vi "sandbox.vi"() -> ()   [LabVIEW 2019, in "Instrument.Lockin.lvlib" / "Instrument UI.Lockin.lvclass"]
uses:
  Instrument UI.Lockin.lvclass
  Instrument.DAQ/Typedefs/State--enum.ctl
  Instrument.DAQ/Instrument.DAQ.lvclass
panel:
  in  "stop":bool
  out "Status":string="Shutdown"
  in  "Enum":T1(ring)=enum."Spinner 3"
  out "delimited string":string
  out "output 1":T2
  # "spinner 3: sweep"
  # "spinner 4: started"
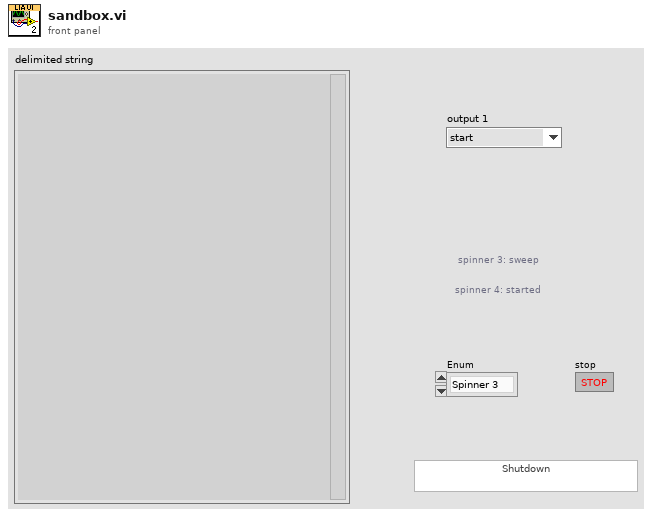
[diagram p1: front panel]
types:
  T1 = enum16{"Spinner 1", "Spinner 2", "Spinner 3", "Spinner 4", "Spinner 5", "Spinner 6"}
  T2 = typedef "Instrument.Lockin.lvlib/Instrument.DAQ.lvclass/State--enum.ctl" = enum16{"start", "stop", "reset", "start sweep", "stop sweep"}
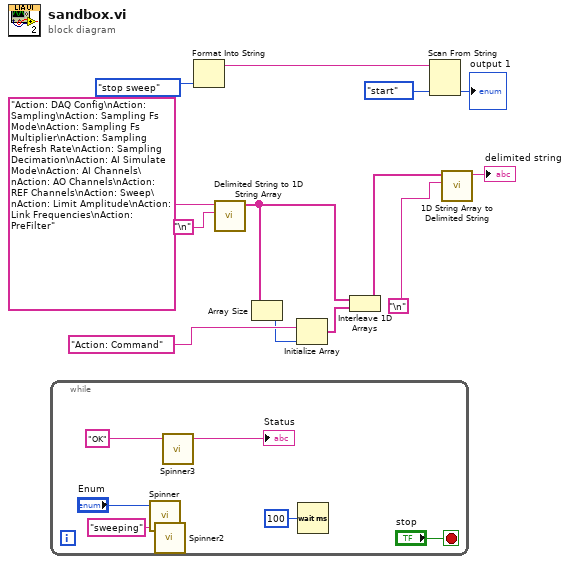
[diagram p0: block diagram]
diagram:
  n1 = while {
    stop <- "stop" stop-if-true
    n2 = call "Spinner.vi"("Enum"="Enum") -> ()  [unwired: 4 in, 1 out]
    n3 = call "Spinner2.vi"("String In"="sweeping") -> ()  [unwired: 4 in, 1 out]
    n4 = call "Spinner3.vi"("String In"="OK") -> ("Spinner Out"=→"Status":string)  [unwired: 4 in]
    n5 = Wait (ms)(milliseconds to wait=u32 100) -> ()  [unwired: 1 out]
  }
  n6 = Format Into String(State--enum."stop sweep" ("State")) -> (resulting string=w11:string)  [unwired: 3 in, 1 out]
  n7 = call <vilib>:"Delimited String to 1D String Array.vi"("delimiter"="\n", "delimited string"="Action: DAQ Config\nAction: Sampling\nAction: Sampling Fs Mode\nAction: Sampling Fs Multiplier\nAction: Sampling Refresh Rate\nAction: Sampling Decimation\nAction: AI Simulate Mode\nAction: AI Channels\nAction: AO Channels\nAction: REF Channels\nAction: Sweep\nAction: Limit Amplitude\nAction: Link Frequencies\nAction: PreFilter" ("State(s) in Front (\"\")")) -> ("string array"=w3:string[])  [unwired: 9 in]
  n8 = Array Size(array=w3) -> (size(s)=w6:i32)
  n9 = Initialize Array("Action: Command", w6) -> (w5:string[])
  n10 = Interleave 1D Arrays(w3, w5) -> (w4:string[])
  n11 = Scan From String(input string=w11, default 1=State--enum."start" ("State")) -> (output 1=→"output 1":T2)  [unwired: 3 in, 3 out]
  n12 = call <vilib>:"1D String Array to Delimited String.vi"("delimiter"="\n", "string array"=w4) -> ("delimited string"=→"delimited string":string)  [unwired: 9 in]
